vi "Query servo for actual status.vi"(8 "error in (no error)":errorcluster, 11 "connection in":variant) -> (0 "error out":errorcluster, 2 "Servo variables":T1, 3 "connection out":variant)   [LabVIEW 2017, in "Servo drive module.lvlib"]
doc: "Query position, target reached and status."
uses:
  Servo drive module.lvlib
  ctl/Servo variables.ctl
  <vilib>/addons/eal4LabVIEW/eal4LabVIEW.lvlib
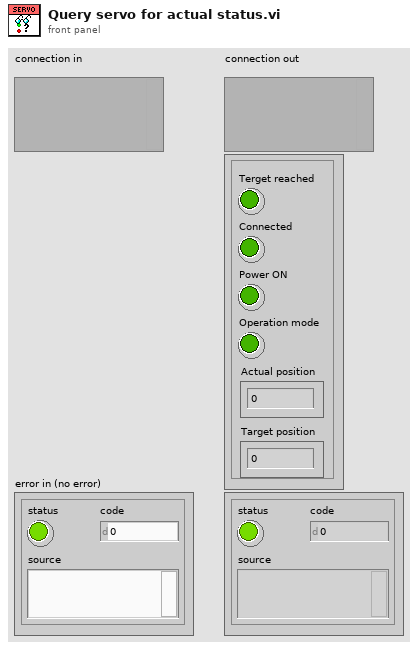
[diagram p1: front panel]
types:
  T1 = typedef "Servo drive module.lvlib/Servo variables.ctl" = cluster{"Terget reached":bool, "Connected":bool, "Power ON":bool, "Operation mode":bool, "Actual position":dbl, "Target position":dbl}
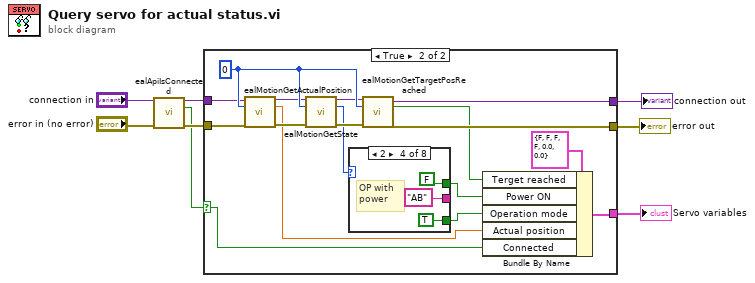
[diagram p0: block diagram]
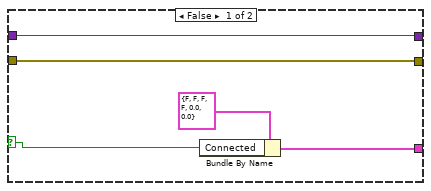
[diagram p2: hidden frame]
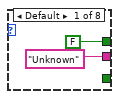
[diagram p3: hidden frame]
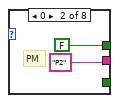
[diagram p4: hidden frame]
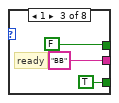
[diagram p5: hidden frame]
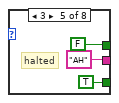
[diagram p6: hidden frame]
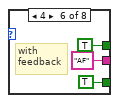
[diagram p7: hidden frame]
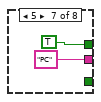
[diagram p8: hidden frame]
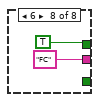
[diagram p9: hidden frame]
diagram:
  n1 = call <vilib>:"ealApiIsConnected.vi"("connection in"="connection in", "error in (no error)"="error in (no error)") -> ("connection out"=w4:variant, "is connected"=w1:bool, "error out"=w3:errorcluster)  [unwired: 11 in]
  n2 = case shown="True" w1 {
    selector: w1 -> [w11 w14]
    tunnel: [w10 w29] -> w7
    tunnel: [w12 w27] -> w6
    tunnel: [w9 w26] -> w5
    tunnel: w4 -> [w9 w16]
    tunnel: w3 -> [w10 w15]
    frame False {
      n3 = Bundle By Name(cluster=T1 {"Terget reached"=FALSE, "Connected"=FALSE, "Power ON"=FALSE, "Operation mode"=FALSE, "Actual position"=0.0, "Target position"=0.0} ("Servo variables"), "Connected"=w11) -> (w12:T1)
    }
    frame True {
      w30 = 0 ("slave index")
      n4 = call <vilib>:"ealMotionGetActualPosition.vi"("connection in"=w16, "slave index"=w30, "error in (no error)"=w15) -> ("connection out"=w17:variant, "getActualPosition"=w19:dbl, "error out"=w24:errorcluster)  [unwired: 10 in]
      n5 = call <vilib>:"ealMotionGetState.vi"("connection in"=w17, "slave index"=w30, "error in (no error)"=w24) -> ("connection out"=w20:variant, "get state"=w21:i32, "error out"=w25:errorcluster)  [unwired: 10 in]
      n6 = case shown="2" w21 {
        tunnel: ["Unknown" "P2" "BB" "AB" "AH" "AF" "PC" "FC"] -> _
        tunnel: [FALSE FALSE FALSE FALSE FALSE TRUE TRUE TRUE] -> w22
        tunnel: [_ _ TRUE TRUE TRUE TRUE _ _] -> w23
        frame Default {
        }
        frame 0 {
          # "PM"
        }
        frame 1 {
          # "ready"
        }
        frame 2 {
          # "OP with\npower"
        }
        frame 3 {
          # "halted"
        }
        frame 4 {
          # "with\nfeedback"
        }
        frame 5 {
        }
        frame 6 {
        }
      }
      n7 = call <vilib>:"ealMotionGetTargetPosReached.vi"("connection in"=w20, "slave index"=w30, "error in (no error)"=w25) -> ("connection out"=w26:variant, "target position reached"=w28:bool, "error out"=w29:errorcluster)  [unwired: 10 in]
      n8 = Bundle By Name(cluster=T1 {"Terget reached"=FALSE, "Connected"=FALSE, "Power ON"=FALSE, "Operation mode"=FALSE, "Actual position"=0.0, "Target position"=0.0} ("Servo variables"), "Terget reached"=w28, "Power ON"=w22, "Operation mode"=w23, "Actual position"=w19, "Connected"=w14) -> (w27:T1)
    }
  }
  "error out" <- w7
  "Servo variables" <- w6
  "connection out" <- w5
